vi "Get PID Angle Gains.vi"(11 "arm in":refnum<class "arm.lvclass">) -> (2 "PID Arm Angle Gains":T1={"proportional gain (Kc)"=1.0, "integral time (Ti, min)"=0.005, "derivative time (Td, min)"=0.0}, 3 "arm out":refnum<class "arm.lvclass">)   [LabVIEW 2015, in "arm.lvclass"]
uses:
  arm.lvclass
  arm.lvclass/arm.ctl
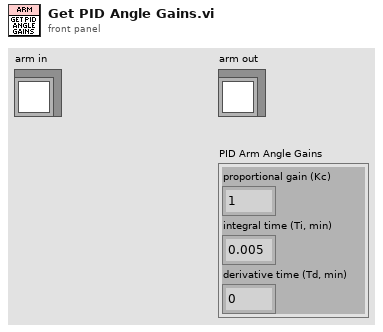
[diagram p1: front panel]
types:
  T1 = cluster{"proportional gain (Kc)":dbl, "integral time (Ti, min)":dbl, "derivative time (Td, min)":dbl}
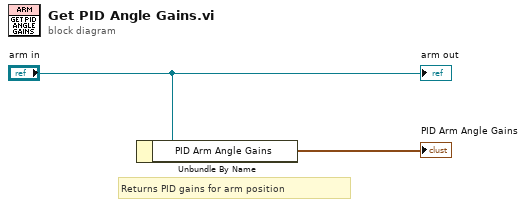
[diagram p0: block diagram]
diagram:
  # "Returns PID gains for arm position"
  n1 = Unbundle By Name("arm in") -> ("PID Arm Angle Gains"=→"PID Arm Angle Gains":T1)
  "arm out" <- "arm in"
